vi "Example_Download_LVHTTPClient.vi"() -> ()   [LabVIEW 2018, in "HttpExamples.lvlib"]
uses:
  HttpExamples.lvlib
  <vilib>/httpClient/LabVIEWHTTPClient.lvlib
panel:
  out "body 2":string
  out "headers 2":string
  out "trimmed string":string
  out "body":string
  out "headers":string
  out "error out":errorcluster
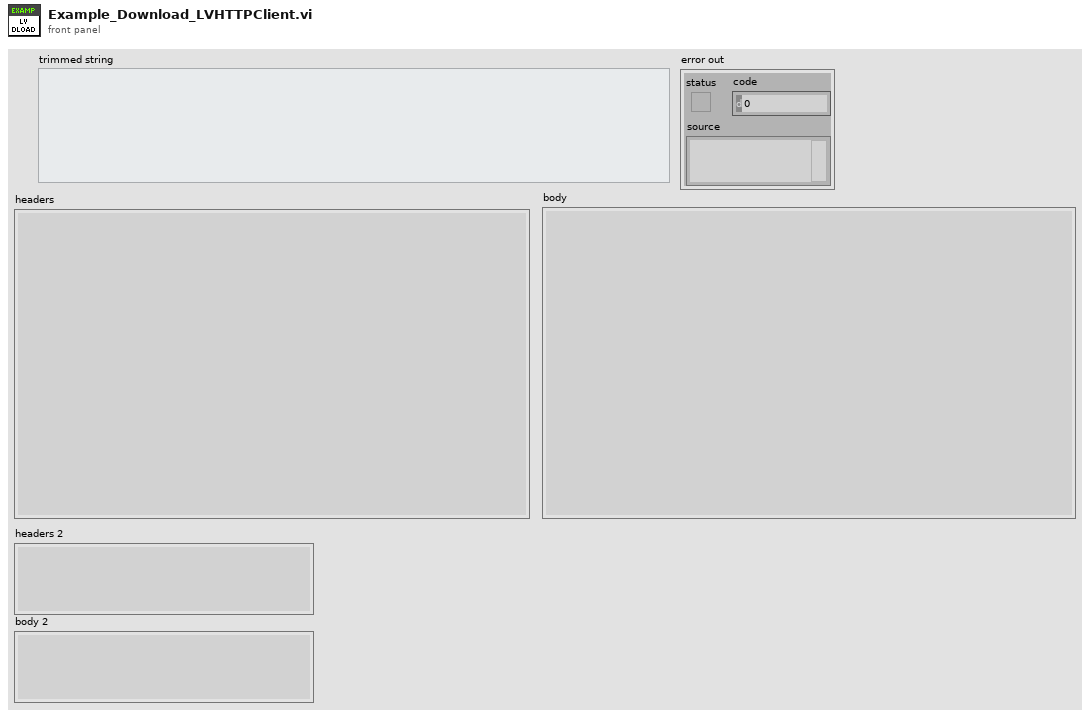
[diagram p1: front panel]
types:
  T1 = typedef "LabVIEWHTTPClient.lvlib/ClientHandle.ctl" = refnum<k1>
  T2 = cluster{"trimmed string":string, "trimmed string":string}
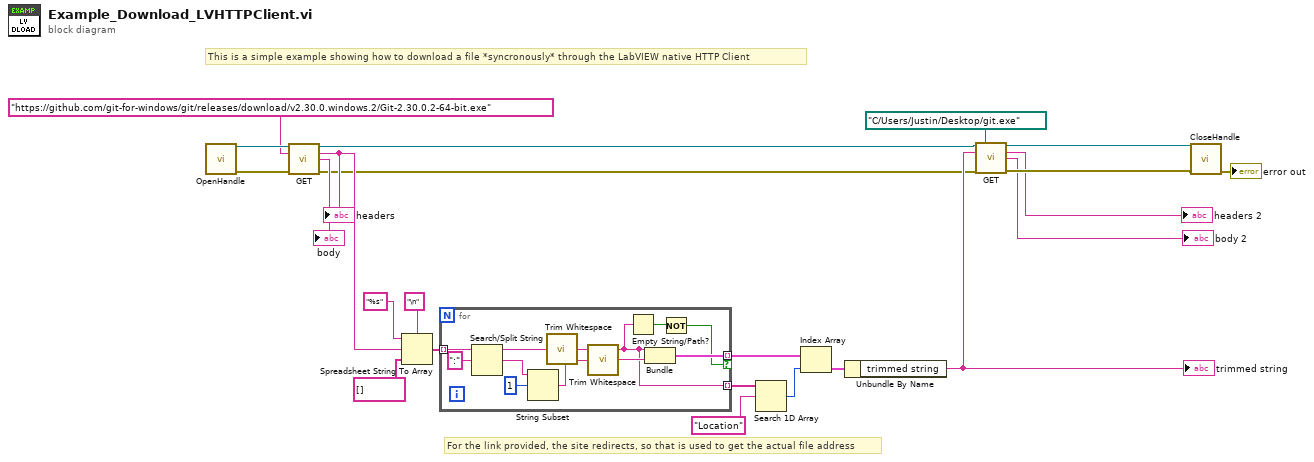
[diagram p0: block diagram]
diagram:
  # "For the link provided, the site redirects, so that is used to get the actual file address"
  # "This is a simple example showing how to download a file *syncronously* through the LabVIEW native HTTP Client"
  n1 = call <vilib>:"OpenHandle.vi"() -> ("client handle out"=w23:T1, "error out"=w22:errorcluster)  [unwired: 14 in]
  n2 = call <vilib>:"GET.vi"("client handle"=w23, "url"="https://github.com/git-for-windows/git/releases/download/v2.30.0.windows.2/Git-2.30.0.2-64-bit.exe", "error in (no error)"=w22) -> ("client handle out"=w7:T1, "headers"=w14:string, "body"=→"body":string, "error out"=w6:errorcluster)  [unwired: 9 in]
  "headers" <- w14
  n3 = Spreadsheet String To Array(delimiter (Tab)="\n", format string="%s", spreadsheet string=w14, array type (2D Dbl)=string[] []) -> (array=w15:string[])
  n4 = for {
    tunnel: w15 -> [w34] mode=indexing
    tunnel: [w31] -> w11 mode=indexing if=w26
    tunnel: [w24] -> w13 mode=indexing
    n5 = Search/Split String(string=w34, search string/char (-)=":") -> (substring before match=w25:string, match + rest of string=w30:string)  [unwired: 1 in, 1 out]
    n6 = String Subset(string=w30, offset (0)=1) -> (substring=w28:string)  [unwired: 1 in]
    n7 = call <vilib>:"Trim Whitespace.vi"("string"=w25) -> ("trimmed string"=w24:string)  [unwired: 1 in]
    n8 = call <vilib>:"Trim Whitespace.vi"("string"=w28) -> ("trimmed string"=w32:string)  [unwired: 1 in]
    n9 = Empty String/Path?(string/path=w24) -> (empty?=w27:bool)
    n10 = Bundle("trimmed string"=w24, "trimmed string"=w32) -> (w31:T2)  [unwired: 1 in]
    n11 = Not(x=w27) -> (.not. x?=w26:bool)
  }
  n12 = Search 1D Array(1D array=w13, element="Location") -> (index of element=w10:i32)  [unwired: 1 in]
  n13 = Index Array(array=w11, index=w10) -> (element=w9:T2)
  n14 = Unbundle By Name(w9) -> ("trimmed string"=w8:string)
  "trimmed string" <- w8
  n15 = call <vilib>:"GET.vi"("client handle"=w7, "output file"=path "C:/Users/Justin/Desktop/git.exe", "url"=w8, "error in (no error)"=w6) -> ("client handle out"=w4:T1, "headers"=→"headers 2":string, "body"=→"body 2":string, "error out"=w5:errorcluster)  [unwired: 8 in]
  n16 = call <vilib>:"CloseHandle.vi"("client handle"=w4, "error in (no error)"=w5) -> ("error out"=→"error out":errorcluster)  [unwired: 13 in]
